vi "timestamp_reversion.vi"(7 "error in (no error)":errorcluster, 10 "Integer Timestamp":i64) -> (0 "error out":errorcluster, 3 "time stamp":timestamp)   [LabVIEW 2012]
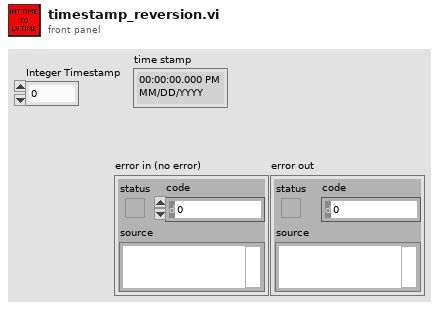
[diagram p1: front panel]
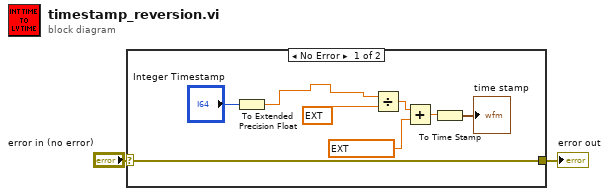
[diagram p0: block diagram]
diagram:
  n1 = case shown="No Error" "error in (no error)" {
    selector: "error in (no error)" -> [w10 w11]
    tunnel: [w10 w11] -> w1
    frame No Error {
      n2 = To Extended Precision Float(1:"Integer Timestamp") -> (0:w5:ext)
      n3 = Divide(x=w5, y=ext 1000.0) -> (x/y=w4:ext)
      n4 = Add(x=w4, y=ext 2082844800.0) -> (x+y=w3:ext)
      n5 = To Time Stamp(1:w3) -> (0:→"time stamp":timestamp)
    }
    frame Error {
    }
  }
  "error out" <- w1
